vi "Sensor Type Lookup.vi"(1 "AI.MeasType":i32(ring)=10300 items=["Voltage"=10322, "Current"=10134, "More:Voltage:Custom with Excitation"=10323, "Frequency"=10181, "Resistance"=10278, "Temperature:Thermocouple"=10303, "Temperature:Thermistor"=10302, "Temperature:RTD"=10301, "Temperature:Built-in Sensor"=10311, "Strain Gage"=10300, "Position:LVDT"=10352, "Position:RVDT"=10353, "Accelerometer"=10356, "Sound Pressure:Microphone"=10354, "TEDS Sensor"=12531]) -> (0 "String Rep":string)   [LabVIEW 2013]
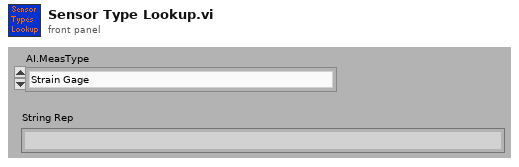
[diagram p1: front panel]
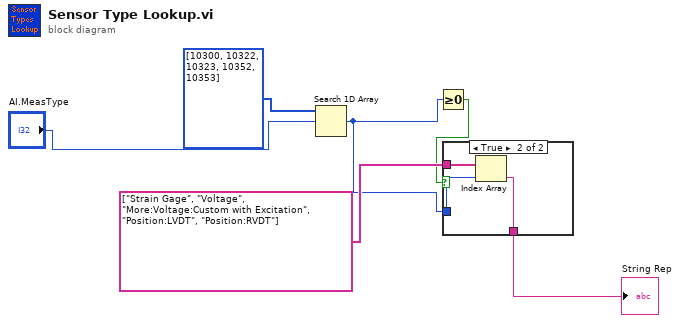
[diagram p0: block diagram]
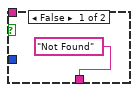
[diagram p2: hidden frame]
diagram:
  n1 = Search 1D Array(1D array=i32[] [10300, 10322, 10323, 10352, 10353], element="AI.MeasType") -> (index of element=w2:i32)  [unwired: 1 out]
  n2 = Greater Or Equal To 0?(x=w2) -> (x >= 0?=w1:bool)
  n3 = case shown="True" w1 {
    tunnel: string[] ["Strain Gage", "Voltage", "More:Voltage:Custom with Excitation", "Position:LVDT", "Position:RVDT"] -> [_ w10]
    tunnel: ["Not Found" w9] -> w3
    tunnel: w2 -> [_ w8]
    frame False {
    }
    frame True {
      n4 = Index Array(array=w10, index=w8) -> (element=w9:string)
    }
  }
  "String Rep" <- w3
